vi "Parallel_FFT_Speed_Test.vi"() -> ()   [LabVIEW 2018]
uses:
  <vilib>/measure/NI_MABase.lvlib
panel:
  out "elapsed":u32
  out "Waveform Graph":dbl[][](graph)
  out "appended array":dbl[][](array[numeric])
  in  "sampling info":cluster{"Fs":dbl, "#s":dbl}={"Fs"=1000.0, "#s"=1000.0} {"Fs" format="%.2p"}
  in  "frequency":dbl=10.0 format="%0.2p"
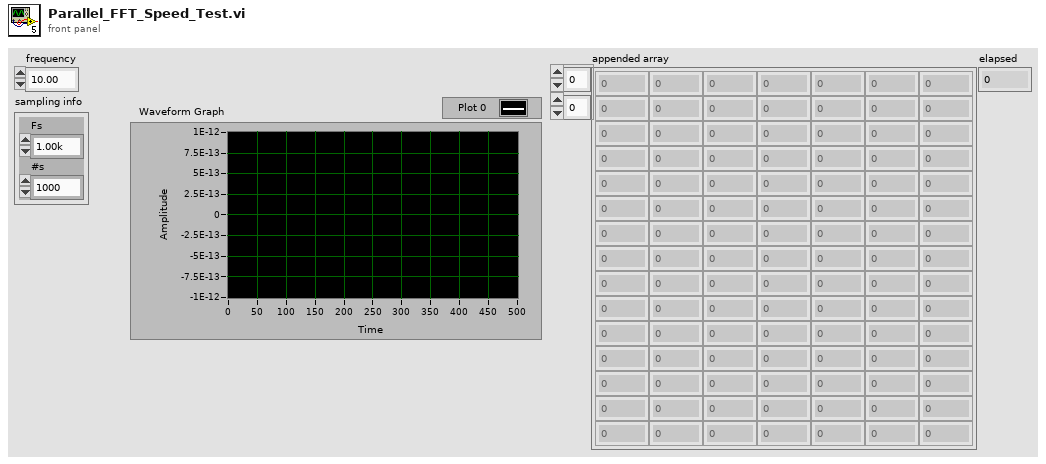
[diagram p1: front panel]
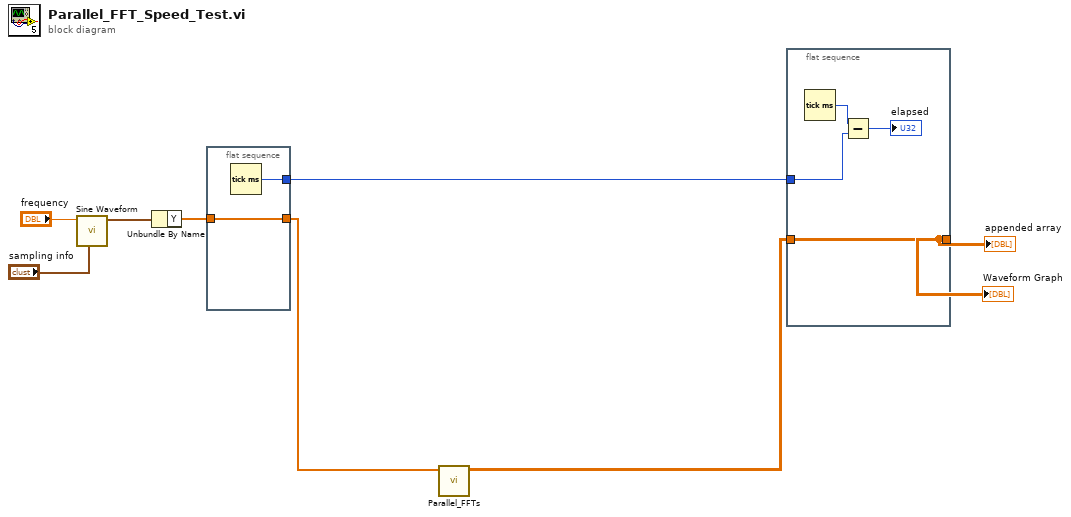
[diagram p0: block diagram]
diagram:
  n1 = call <vilib>:"Sine Waveform.vi"("sampling info"="sampling info", "frequency"="frequency") -> ("signal out"=w6:waveform(dbl))  [unwired: 8 in, 1 out]
  n2 = Unbundle By Name(w6) -> ("Y"=w4:dbl[])
  n3 = flat-sequence {
    tunnel: [w10] -> w5
    tunnel: w4 -> [w10]
    tunnel: [w9] -> w1
    frame #0 {
      n4 = Tick Count (ms)() -> (millisecond timer value=w9:u32)
    }
  }
  n5 = call "Parallel_FFTs.vi"("Y"=w5) -> ("10 Hz FFTs"=w3:dbl[][])  [unwired: 9 in, 1 out]
  n6 = flat-sequence {
    tunnel: [w14] -> w2
    tunnel: w3 -> [w14]
    tunnel: w1 -> [w11]
    frame #0 {
      n7 = Tick Count (ms)() -> (millisecond timer value=w13:u32)
      n8 = Subtract(x=w13, y=w11) -> (x-y=→"elapsed":u32)
    }
  }
  "appended array" <- w2
  "Waveform Graph" <- w2
